vi "getGain.vi"(8 "error in (no error)":errorcluster, 11 "OptCtrl in":refnum<class "OptCtrl.lvclass">) -> (0 "error out":errorcluster, 2 "Gain":dbl, 3 "OptCtrl out":refnum<class "OptCtrl.lvclass">)   [LabVIEW 2016, in "OptCtrl.lvclass"]
uses:
  OptCtrl.lvclass
  OptCtrl.lvclass/OptCtrl.ctl
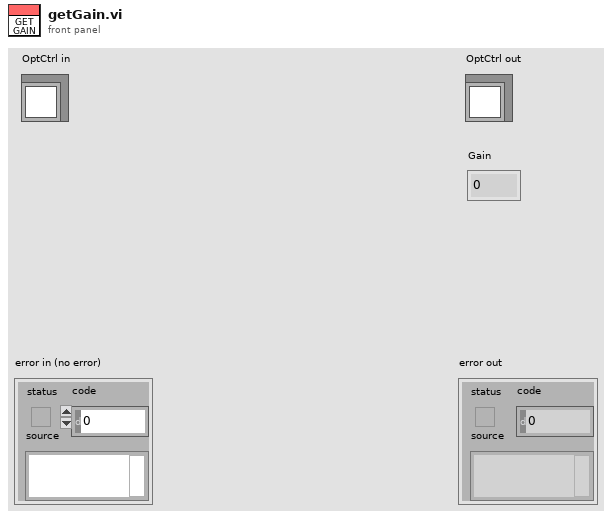
[diagram p1: front panel]
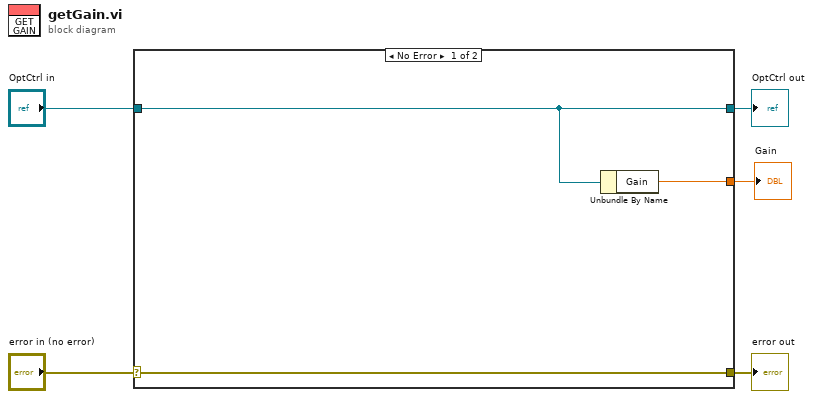
[diagram p0: block diagram]
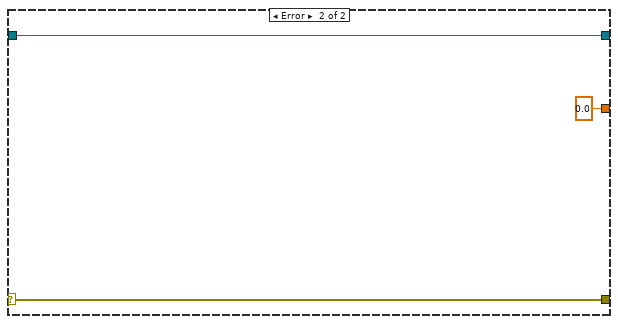
[diagram p2: hidden frame]
diagram:
  n1 = case shown="No Error" "error in (no error)" {
    selector: "error in (no error)" -> [w8 w11]
    tunnel: [w8 w11] -> w4
    tunnel: [w7 w10] -> w2
    tunnel: "OptCtrl in" -> [w7 w10]
    tunnel: [w6 0.0 ("Gain")] -> w1
    frame No Error {
      n2 = Unbundle By Name(w7) -> ("Gain"=w6:dbl)
    }
    frame Error {
    }
  }
  "error out" <- w4
  "OptCtrl out" <- w2
  "Gain" <- w1
